vi "Thermometer.vi"(1 "단위 (0: 섭씨)":u16(ring) items=["섭씨", "화씨"]) -> (0 "온도":dbl(slide) scale=0.0..100.0)   [LabVIEW 2018]
doc: "이 VI는 DAQ BNC-2120 터미널 블록의 온도 센서를 사용하여 온도를 측정합니다."
uses:
  Instance           1 19Saved   Thermometer .vi
  Instance           2 19Saved   Thermometer .vi
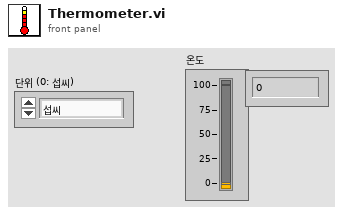
[diagram p1: front panel]
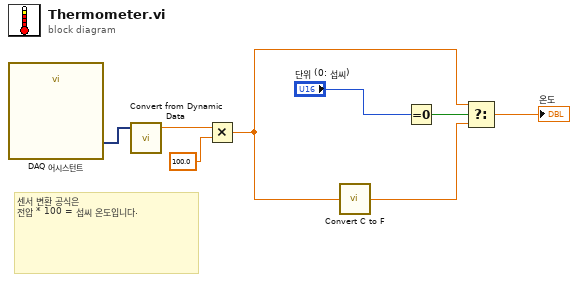
[diagram p0: block diagram]
diagram:
  # "센서 변환 공식은 \n전압 * 100 = 섭씨 온도입니다."
  n1 = call "DAQ 어시스턴트"() -> ("data"=w7:dynamicdata)  [unwired: 17 in, 2 out]
  n2 = call "Convert from Dynamic Data"("Dynamic Data Type"=w7) -> ("Scalar"=w5:dbl)  [unwired: 3 in]
  n3 = Multiply(x=w5, y=100.0) -> (x*y=w6:dbl)
  n4 = call "Convert C to F.vi"("섭씨 온도"=w6) -> ("화씨 온도"=w8:dbl)
  n5 = Equal To 0?(x="단위 (0: 섭씨)") -> (x = 0?=w1:bool)
  n6 = Select(t=w6, s=w1, f=w8) -> (s? t:f=→"온도":dbl)
